vi "Read Analog Inputs.vi"(11 "VISA Refnum in":refnum<visa-resource-name>) -> (0 "error out":errorcluster, 2 "Analog Inputs":u16[](array[numeric]), 3 "VISA Refnum out":refnum<visa-resource-name>)   [LabVIEW 2020, in "RaspberryPiPico.lvlib"]
uses:
  RaspberryPiPico.lvlib
  <instrlib>/HandsOnPi2040/Public/AnaIns.ctl
  <instrlib>/HandsOnPi2040/HandsOnPi2040.lvlib
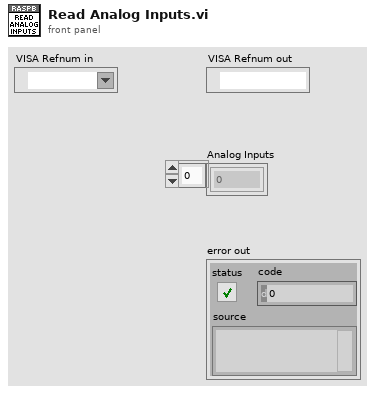
[diagram p1: front panel]
types:
  T1 = typedef "HandsOnPi2040.lvlib/AnaIns.ctl" = enum16{"No AI - Error", "AI1 (GPIO26)", "AI2 (GPIO27)"}
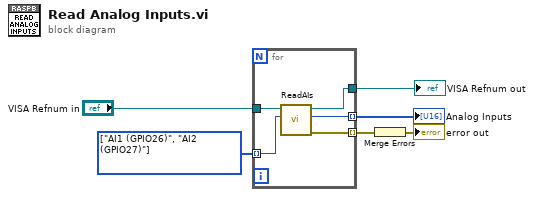
[diagram p0: block diagram]
diagram:
  w2 = T1[] [enum."AI1 (GPIO26)", enum."AI2 (GPIO27)"] items=["No AI - Error", "AI1 (GPIO26)", "AI2 (GPIO27)"] ("Array")
  n1 = for {
    tunnel: "VISA Refnum in" -> [w10]
    tunnel: [w9] -> w5
    tunnel: w2 -> [w8] mode=indexing
    tunnel: [w7] -> w4 mode=indexing
    tunnel: [w11] -> w3 mode=indexing
    n2 = call <instrlib>:"ReadAIs.vi"("Analog Inputs"=w8, "VISA resource name"=w10) -> ("error out"=w11:errorcluster, "Value"=w7:u16, "VISA resource name out"=w9:refnum<visa-resource-name>)  [unwired: 7 in]
  }
  "VISA Refnum out" <- w5
  "Analog Inputs" <- w4
  n3 = Merge Errors(w3) -> (→"error out":errorcluster)
